vi "List Compatible Ctls.vi"(11 "UIP In":refnum<class "UIP Interface.lvclass">) -> (2 "Compatible Ctl Classes":string[](array[string]), 3 "UIP Out":refnum<class "UIP Interface.lvclass">)   [LabVIEW 2020, in "UIM.lvlib" / "UIP Interface.lvclass"]
doc: "Overwrite this method in your child UIPs to provide a custom list of VI Server Control Classes compatible with that UIP."
uses:
  UIP Interface/UIP Interface.lvclass
panel:
  in  "Numeric Ctl":dbl
  # "These are controls compatible \nwith your UIP. Use them as\nhelpers to extract class names\nfrom references."
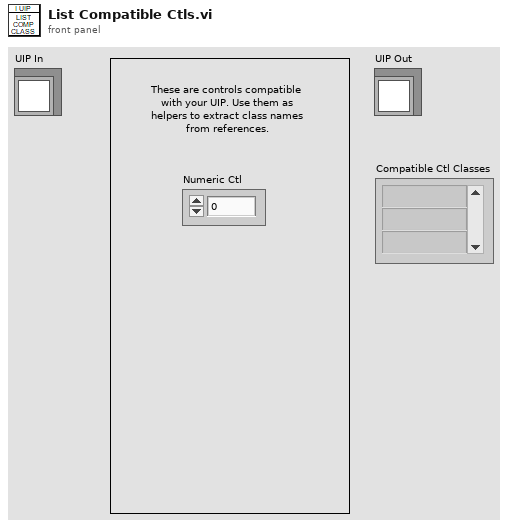
[diagram p1: front panel]
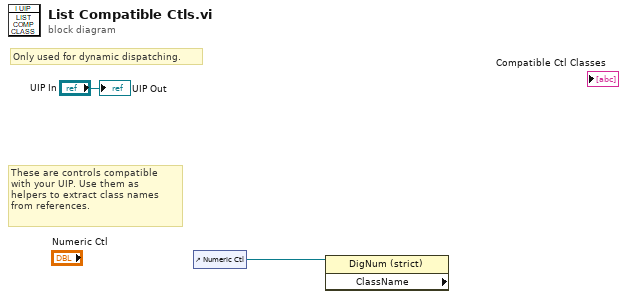
[diagram p0: block diagram]
diagram:
  # "These are controls compatible \nwith your UIP. Use them as\nhelpers to extract class names\nfrom references."
  # "Only used for dynamic dispatching."
  n1 = control-ref of="Numeric Ctl"() -> (w1:refnum<vi>)
  n2 = property class="DigNum (strict)" props=["ClassName"](reference=w1) -> ()  [unwired: 1 in, 3 out]
  "UIP Out" <- "UIP In"
